vi "FITS - Save Multiple Images to FITS.vi"(5 "NAXIS":string="4", 6 "Neo Info":T1={"Handle"=104, "Pixel Encoding"="Mono16", "AOI Width"=2560, "AOI Height"=2160, "AOI Stride"=5136, "Row Readout Time"=9.371428571428572e-06, "Frame Readout Time"=0.010121142857142858, "Interframe Time"=8.434285714285715e-05, "Semaphore"=refnum, "SerialNumber"="SCC-02209", "Camera Model"="DC-152Q-C00-FI", "Controller ID"="3", "Firmware Version"="13.8.26.122", "Shutter"="Global", "BDiv"=1, "Time at Synch"=timestamp(3029526000.379448 s since 1904-01-01), "Idx"=0, "PreAmp"="", "Binning"=enum."1x1", "PixelReadoutRate"="", "Exposure (s)"=0.05, "Image Bytes"=11098896, "Image Pixels"=5529600, "SpuriousNoiseFilter"=FALSE, "Overlap"=FALSE, "CycleMode"=""} {"Exposure (s)" format="%^.3g"; "Time at Synch" format="%<%H:%M:%S>T"; "Interframe Time" format="%#_3g"; "Frame Readout Time" format="%_3g"; "Row Readout Time" format="%_3g"}, 7 "FITS Header":T4={"Wavelength (nm)"=530.15, "Exposure (s)"=0.05, "Tuning Delay (ms)"=1000.0, "Beam Type (-1/1)"=1.0, "Tuning Voltages"=[1.111, 2.222, 3.333, 4.444], "Observer"="observer", "Light Shapping Diffuser"=enum."In Beam", "Comment"="", "Data Type"=enum."HOLE", "Mod Cycles"=0, "SCD Calibration Optics"=enum."1 - Polarizer @0, I+Q", "SCD Emission Line Filter"=enum."1-557.6nm", "Cookbook"="", "COMP-S Calibration Wheel"=enum."Dark", "COMP-S Andover Filter Wheel"=enum."530.3nm/HWB 0.34nm (Fe XIV)", "FOV Rotation (deg)"=66.0, "Objective Lens Position (mm)"=0.0, "Occulter size"=0.0, "Time End"=timestamp(3382374145.421875 s since 1904-01-01), "Acc Exposure (s)"=0.0, "Time Stamp Array"=[], "Camera Serial Number"=[], "Camera Temp"=[], "Camera PI (mm)"=[], "Time Start"=timestamp(3382374145.421875 s since 1904-01-01), "Peripherals"={"ILX controler"=FALSE, "Zone temperatures"=FALSE, "Andor"=FALSE, "Andor 2"=FALSE, "PI Stages"=FALSE, "AISAS mechanisms"=FALSE, "AISAS Mech.lvclass"=refnum, "Zone temp ref"=variant, "FWs"=FALSE}, "FITS paths"=[], "Cameras"=enum."Andor", "load preset cbk"=FALSE, "periodic check count"=0, "COMP-S Calibration Wheel 2"=enum."Dark", "Calib"=enum."Dark", "Abso Aperture"=66.0, "Nominal Aperture"=66.0} {"Nominal Aperture" format="%.1f"; "Abso Aperture" format="%.1f"; "Camera PI (mm)" format="%_3g"; "Acc Exposure (s)" format="%^.3g"; "Occulter size" format="%.2f"; "Objective Lens Position (mm)" min=70.0 max=152.0 format="%.2f"; "FOV Rotation (deg)" format="%.1f"; "Exposure (s)" format="%^.3g"; "Wavelength (nm)" format="%_6g"}, 8 "error in":errorcluster, 9 "I32 Image Data":i32[](array[numeric]), 10 "Image #":i32, 11 "FITS File Path":path=path "G:/SCD Data/Level-0/20141030/20141030.160747.FTS") -> (0 "error out":errorcluster, 2 "FITS Write Time (ms)":u32, 3 "FITS Path Out":path=path "G:/SCD Data/Level-0/20141030/20141030.160747.FTS")   [LabVIEW 2014]
doc: "Duplicate first measurement\nand put it in first element of\nmeasurement array. This\nis a dummy measurement for the\nprimary header. This is because\nwe don't want any images associated\nwith the primary HDU, just the \nextensions. In the Make FITS\nHeaders VI, the NAXIS is set to 0 in\nthis primary HDU"
uses:
  Controls/SCD - FITS Cluster.ctl
  AISAS/Mech/AISAS Mech.lvclass
  AISAS/Controls/Diffuser.ctl
  Controls/FITS Data type.ctl
  Controls/SCD - Calibration Optics Filter Wheel.ctl
  Controls/SCD - EDT - Emission Line Filter Wheel.ctl
  Controls/CoMP-S Controls/Polarization Optics Filter Wheel.ctl
  Controls/CoMP-S Controls/Emission Line Filter Wheel.ctl
  AISAS/Controls/focus.ctl
  Controls/peripherals.ctl
  Controls/Cameras select.ctl
  Camera/Andor Neo Info.ctl
  Controls/beaning.ctl
panel:
  in  "disable buffering (T)":bool=TRUE
  out "header byte length":i32=23040
  out "sector size (bytes)":u32
  out "size(s)":i32
  # "Useful FITS Information\nhttp://www.digitalpreservation.gov/formats/fdd/fdd000317.shtml\n\nFITS Standard 3 Requirements\n\nData in a FITS file is required to be stored in big-endian byte order.\nI16, I32, I64 are supported as well as DBL Floating Point but not \n(to my knowledge) U16"
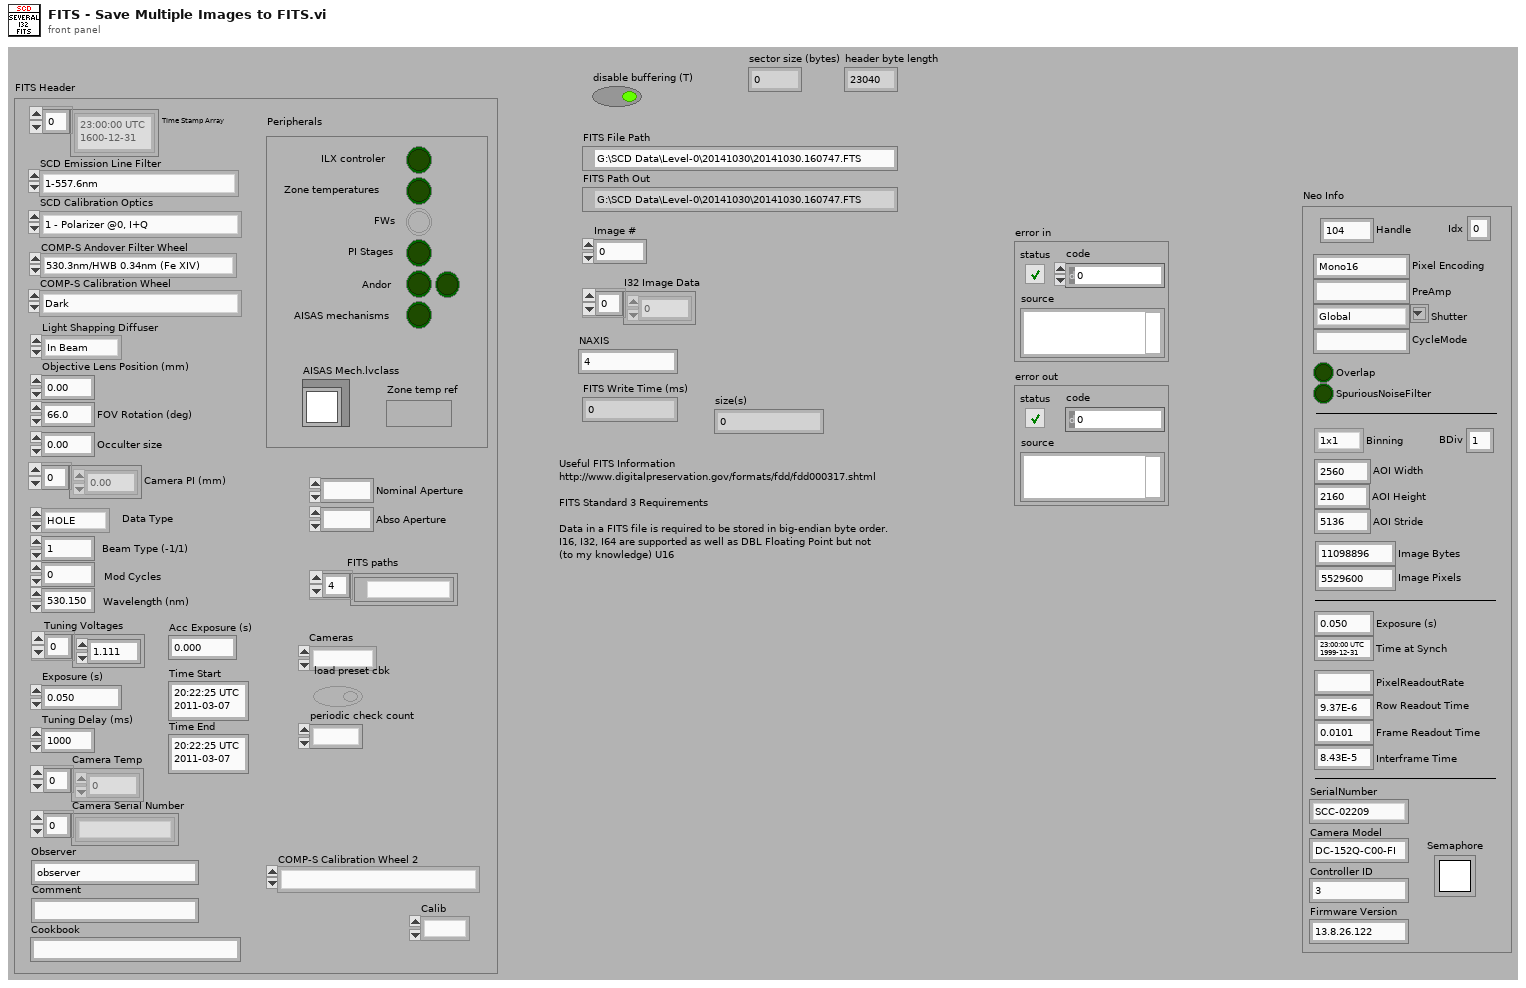
[diagram p1: front panel]
types:
  T1 = typedef "Andor Neo Info.ctl" = cluster{"Handle":i32, "Pixel Encoding":string, "AOI Width":i32, "AOI Height":i32, "AOI Stride":i32, "Row Readout Time":dbl, "Frame Readout Time":dbl, "Interframe Time":dbl, "Semaphore":T2, "SerialNumber":string, "Camera Model":string, "Controller ID":string, "Firmware Version":string, "Shutter":string, "BDiv":u8, "Time at Synch":timestamp, "Idx":i32, "PreAmp":string, "Binning":T3, "PixelReadoutRate":string, "Exposure (s)":dbl, "Image Bytes":i64, "Image Pixels":i64, "SpuriousNoiseFilter":bool, "Overlap":bool, "CycleMode":string}
  T2 = typedef "Semaphore RefNum" = refnum<k1>
  T3 = typedef "beaning.ctl" = enum16{"1x1", "2x2", "3x3", "4x4", "8x8"}
  T4 = typedef "SCD - FITS Cluster.ctl" = cluster{"Wavelength (nm)":dbl, "Exposure (s)":dbl, "Tuning Delay (ms)":dbl, "Beam Type (-1/1)":dbl, "Tuning Voltages":dbl[], "Observer":string, "Light Shapping Diffuser":T5, "Comment":string, "Data Type":T6, "Mod Cycles":u16, "SCD Calibration Optics":T7, "SCD Emission Line Filter":T8, "Cookbook":string, "COMP-S Calibration Wheel":T9, "COMP-S Andover Filter Wheel":T10, "FOV Rotation (deg)":dbl, "Objective Lens Position (mm)":T11, "Occulter size":dbl, "Time End":timestamp, "Acc Exposure (s)":dbl, "Time Stamp Array":timestamp[], "Camera Serial Number":string[], "Camera Temp":dbl[], "Camera PI (mm)":dbl[], "Time Start":timestamp, "Peripherals":T12, "FITS paths":path[], "Cameras":T13, "load preset cbk":bool, "periodic check count":i32, "COMP-S Calibration Wheel 2":T9, "Calib":enum16{"Dark", "Flat"}, "Abso Aperture":dbl, "Nominal Aperture":dbl}
  T5 = typedef "Diffuser.ctl" = enum16{"Out of Beam", "In Beam"}
  T6 = typedef "FITS Data type.ctl" = enum16{"LIVE", "DARK", "FLAT", "CALI", "OBSE", "ABSO", "AURE", "TARG", "OBJE", "HOLE", "OREX", "THRO", "CHIP"}
  T7 = typedef "SCD - Calibration Optics Filter Wheel.ctl" = enum16{"1 - Polarizer @0, I+Q", "2 - Polarizer @90, I-Q", "3 - Polarizer @45, I+U", "4 - Polarizer @135, I-U", "5 - Polarizer @0, Retarder @45, I+V", "6 - Polarizer @0, Retarder @135, I-V", "7 - Dark", "8 - Clear", "9 - N/A"}
  T8 = typedef "SCD - EDT - Emission Line Filter Wheel.ctl" = enum16{"1-557.6nm", "2-587.6nm", "3-589.6nm", "4-630.2nm", "5-656.4nm", "6-849.8nm", "7-854.2nm", "8-866.2nm", "9-1083.0nm"}
  T9 = typedef "Polarization Optics Filter Wheel.ctl" = enum16{"Dark", "Clear", "Exchange Lens", "Polarizer @0, I+Q", "Polarizer @90, I-Q", "Polarizer @45, I+U", "Polarizer @135, I-U", "Polarizer @0, Retarder @45, I+V", "Polarizer @0, Retarder @135, I-V"}
  T10 = typedef "Emission Line Filter Wheel.ctl" = enum16{"530.3nm/HWB 0.34nm (Fe XIV)", "587.6nm/HBW 0.44nm (He I D3)", "637.5nm/HBW 0.53nm (Fe X)", "656.3nm/HBW 0.57nm (H-Alpha)", "789.2nm/HBW 0.85nm (Fe XI)", "854.2nm/HBW 1.01nm (Ca I)", "1074.7nm/HBW 2.34nm (Fe XIII)", "1079.8nm/HBW 1.64nm (Fe XIII)", "1083.0nm/HBW 1.66nm (He I)"}
  T11 = typedef "focus.ctl" = dbl
  T12 = typedef "peripherals.ctl" = cluster{"ILX controler":bool, "Zone temperatures":bool, "Andor":bool, "Andor 2":bool, "PI Stages":bool, "AISAS mechanisms":bool, "AISAS Mech.lvclass":refnum<class "AISAS Mech.lvclass">, "Zone temp ref":variant, "FWs":bool}
  T13 = typedef "Cameras select.ctl" = enum16{"Andor", "GDR"}
  T14 = enum16{"open", "replace", "create", "open or create", "replace or create", "replace or create with confirmation"}
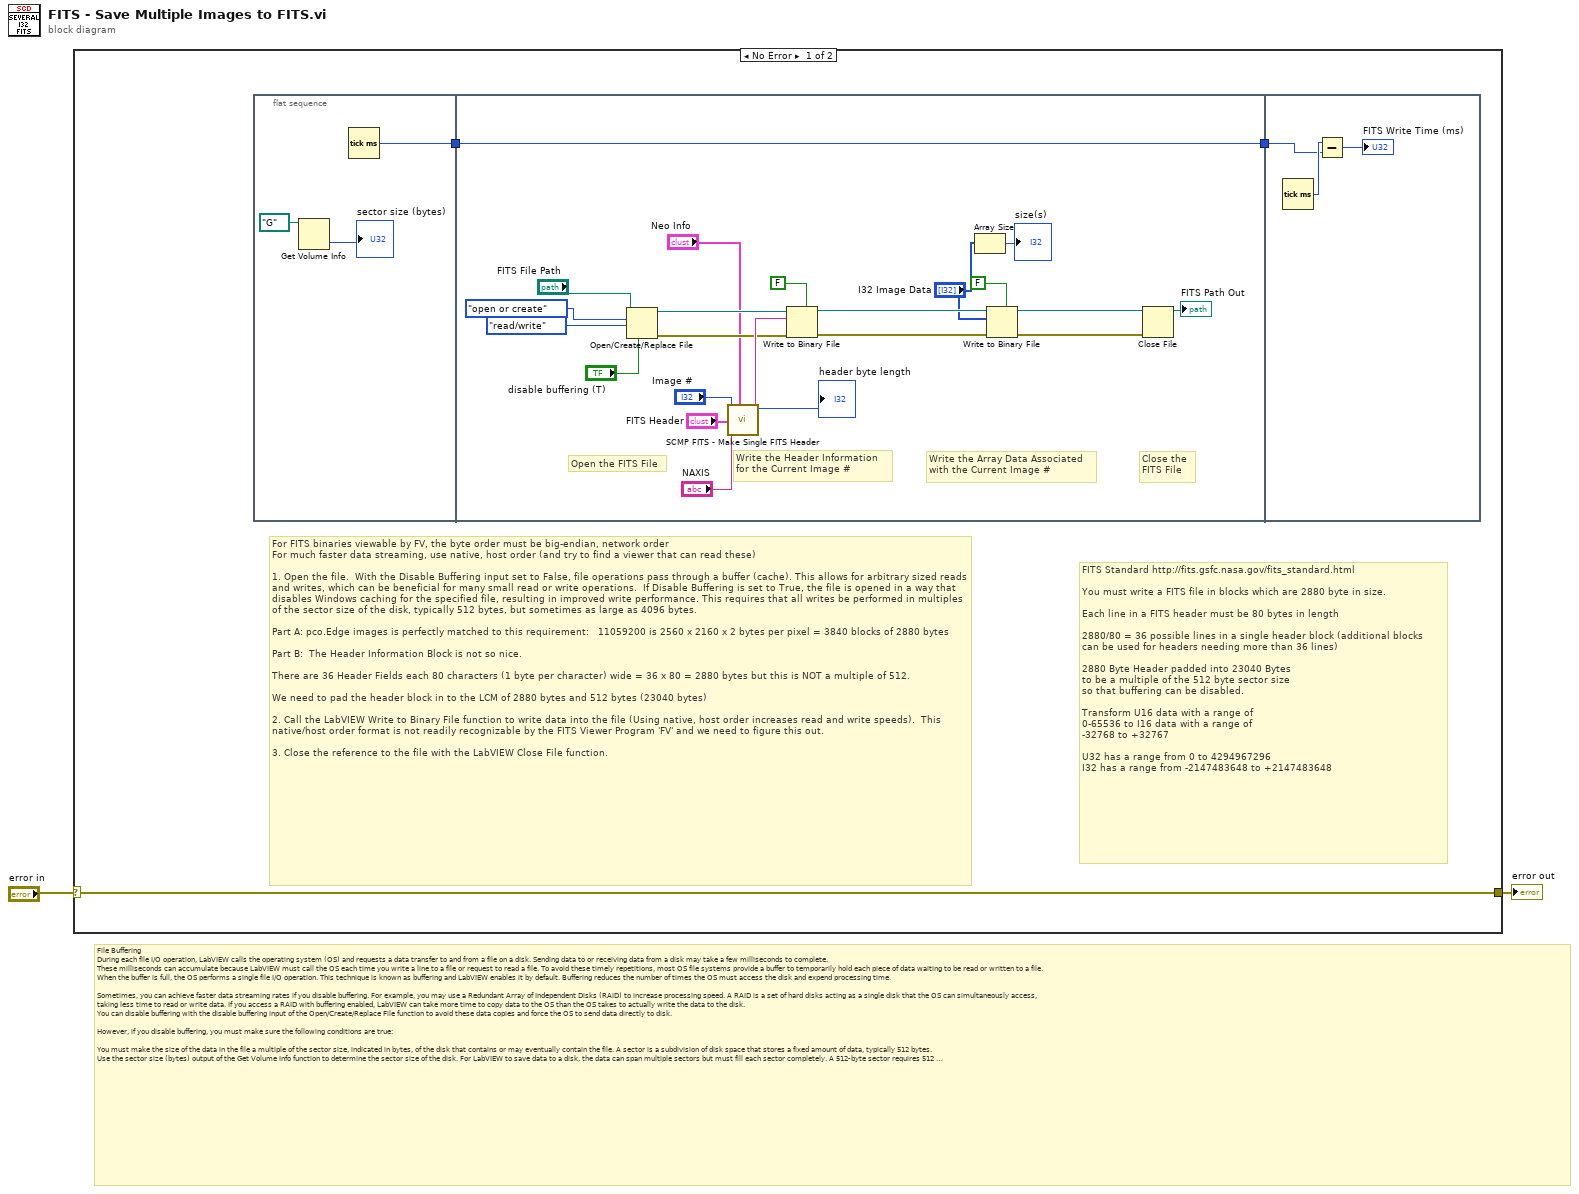
[diagram p0: block diagram]
diagram:
  # "File Buffering\nDuring each file I/O operation, LabVIEW calls the operating system (OS) and requests a data transfer to and from a file on a disk. Sending data to or receiving data from a disk may take a few milliseconds to complete. \nThese milliseconds can accumulate because LabVIEW must call the OS each time you write a line to a file or request to read a file. To avoid these timely repetitions, most OS file systems provide a buffer to temporarily hold each piece of data waiting to be read or written to a file. \nWhen the buffer is full, the OS performs a single file I/O operation. This technique is known as buffering and LabVIEW enables it by default. Buffering reduces the number of times the OS must access the disk and expend processing time. \n\nSometimes, you can achieve faster data streaming rates if you disable buffering. For example, you may use a Redundant Array of Independent Disks (RAID) to increase processing speed. A RAID is a set of hard disks acting as a single disk that the OS can simultaneously access, \ntaking less time to read or write data. If you access a RAID with buffering enabled, LabVIEW can take more time to copy data to the OS than the OS takes to actually write the data to the disk. \nYou can disable buffering with the disable buffering input of the Open/Create/Replace File function to avoid these data copies and force the OS to send data directly to disk.\n\nHowever, if you disable buffering, you must make sure the following conditions are true:\n\nYou must make the size of the data in the file a multiple of the sector size, indicated in bytes, of the disk that contains or may eventually contain the file. A sector is a subdivision of disk space that stores a fixed amount of data, typically 512 bytes. \nUse the sector size (bytes) output of the Get Volume Info function to determine the sector size of the disk. For LabVIEW to save data to a disk, the data can span multiple sectors but must fill each sector completely. A 512-byte sector requires 512 bytes of data. \nIf the data is not a multiple of the sector size, you must pad the data with filler data and delete the filler data before LabVIEW reads back the file. \nThe data in the file must be aligned to a multiple of the alignment the disk requires. LabVIEW aligns the data, and you cannot change that alignment. If the data does not meet the alignment requirement, LabVIEW returns an error and you must enable buffering and reopen the file."
  n1 = case shown="No Error" "error in" {
    selector: "error in" -> [w5 w34]
    tunnel: [w5 w34] -> w1
    frame No Error {
      # "FITS Standard http://fits.gsfc.nasa.gov/fits_standard.html\n\nYou must write a FITS file in blocks which are 2880 byte in size.\n\nEach line in a FITS header must be 80 bytes in length\n\n2880/80 = 36 possible lines in a single header block (additional blocks\ncan be used for headers needing more than 36 lines)\n\n2880 Byte Header padded into 23040 Bytes\nto be a multiple of the 512 byte sector size\nso that buffering can be disabled.\n\nTransform U16 data with a range of\n0-65536 to I16 data with a range of\n-32768 to +32767\n\nU32 has a range from 0 to 4294967296\nI32 has a range from -2147483648 to +2147483648"
      # "For FITS binaries viewable by FV, the byte order must be big-endian, network order\nFor much faster data streaming, use native, host order (and try to find a viewer that can read these)\n\n1. Open the file.  With the Disable Buffering input set to False, file operations pass through a buffer (cache). This allows for arbitrary sized reads and writes, which can be beneficial for many small read or write operations.  If Disable Buffering is set to True, the file is opened in a way that disables Windows caching for the specified file, resulting in improved write performance. This requires that all writes be performed in multiples of the sector size of the disk, typically 512 bytes, but sometimes as large as 4096 bytes.\n\nPart A: pco.Edge images is perfectly matched to this requirement:   11059200 is 2560 x 2160 x 2 bytes per pixel = 3840 blocks of 2880 bytes\n\nPart B:  The Header Information Block is not so nice.  \n\nThere are 36 Header Fields each 80 characters (1 byte per character) wide = 36 x 80 = 2880 bytes but this is NOT a multiple of 512.\n\nWe need to pad the header block in to the LCM of 2880 bytes and 512 bytes (23040 bytes)\n\n2. Call the LabVIEW Write to Binary File function to write data into the file (Using native, host order increases read and write speeds).  This native/host order format is not readily recognizable by the FITS Viewer Program 'FV' and we need to figure this out.\n\n3. Close the reference to the file with the LabVIEW Close File function."
      n2 = flat-sequence {
        tunnel: [w8] -> w3
        tunnel: [w16] -> w4
        tunnel: w3 -> [w16]
        tunnel: w4 -> [w31]
        frame #0 {
          n3 = Get Volume Info(11:path "G:/" ("path")) -> (4:→"sector size (bytes)":u32)  [unwired: 1 in, 5 out]
          n4 = Tick Count (ms)() -> (millisecond timer value=w8:u32)
        }
        frame #1 {
          # "Close the \nFITS File"
          # "Write the Array Data Associated\nwith the Current Image #"
          # "Write the Header Information\nfor the Current Image #"
          # "Open the FITS File"
          n5 = Open/Create/Replace File(file path (use dialog)="FITS File Path", operation (0:open)=T14."open or create", access (0:read/write)=enum16{"read/write", "read-only", "write-only"}."read/write", disable buffering (F)="disable buffering (T)") -> (refnum out=w19:refnum<file>, error out=w20:errorcluster)  [unwired: 1 in, 2 out]
          n6 = call "SCMP FITS - Make Single FITS Header.vi"("Andor"="Neo Info", "NAXIS"="NAXIS", "FITS Header"="FITS Header", "Image #"="Image #") -> ("23040 Byte Header"=w22:string, "final header byte length"=→"header byte length":i32)  [unwired: 2 in, 4 out]
          n7 = Write to Binary File(file (use dialog)=w19, data=w22, error in=w20, 5:FALSE ("prepend array or string size? (T)")) -> (refnum out=w18:refnum<file>, error out=w21:errorcluster)  [unwired: 3 out]
          n8 = Array Size(array="I32 Image Data") -> (size(s)=→"size(s)":i32)
          n9 = Write to Binary File(file (use dialog)=w18, data="I32 Image Data", error in=w21, 5:FALSE ("prepend array or string size? (T)")) -> (refnum out=w29:refnum<file>, error out=w30:errorcluster)  [unwired: 3 out]
          n10 = Close File(refnum=w29, error in=w30) -> (path=→"FITS Path Out":path)  [unwired: 1 out]
        }
        frame #2 {
          n11 = Tick Count (ms)() -> (millisecond timer value=w32:u32)
          n12 = Subtract(x=w32, y=w31) -> (x-y=→"FITS Write Time (ms)":u32)
        }
      }
    }
    frame Error {
    }
  }
  "error out" <- w1
